vi "Read Multiple Sequence.vi"(6 "Segment number (0: All segment)":i16, 8 "error in (no error)":errorcluster, 9 "Timeout (10000 ms)":u32=10000, 10 "Channels":u16[](array[ring])=[0, 1] items=["Channel 1", "Channel 2", "Channel 3", "Channel 4", "Memory 1", "Memory 2", "Memory 3", "Memory 4", "Function 1", "Function 2", "Function 3", "Function 4", "Function 5", "Function 6", "Function 7", "Function 8"], 11 "VISA resource name":refnum<visa-resource-name>) -> (0 "error out":errorcluster, 2 "Waveform Data":waveform(dbl)[](graph), 3 "VISA resource name out":refnum<visa-resource-name>)   [LabVIEW 2013, in "LeCroy Wave Series.lvlib"]
doc: "Initiates an acquisition on all channels that you enabled with the <B>Configure Channel</B> VI. The VI waits for the acquisition to complete and returns the segments of waveform for the Source Channels you specified. If the oscilloscope did not complete the acquisition within the time period you specify with the Timeout parameter, the VI returns a time out error. A common cause for a timeout error is the acquisition was not triggered. For example, the trigger level is out of range of the waveform. \n\nNote: If your instrument does not support auto compensation for probe attenuation, you may need to adjust the scaling of the Waveform Data accordingly. This is handled automatically in the <B>Configure Channel</B> VI or can be done manually by multiplying the Waveform Data by the probe attenuation."
uses:
  LeCroy Wave Series.lvlib
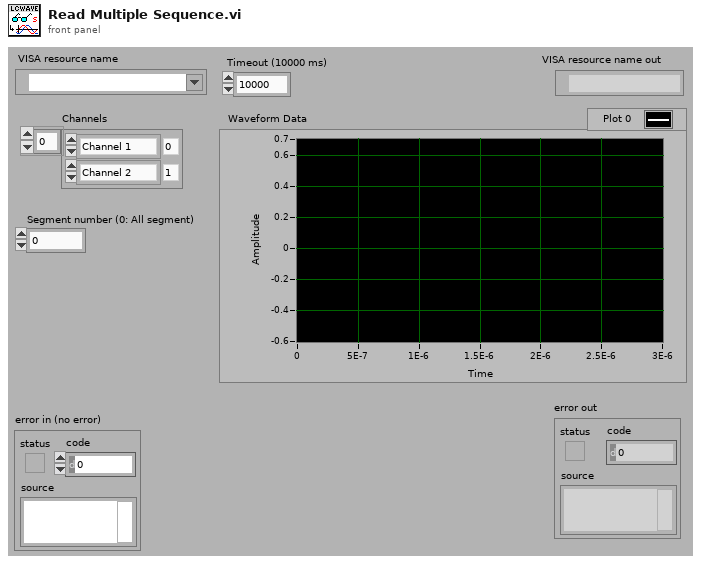
[diagram p1: front panel]
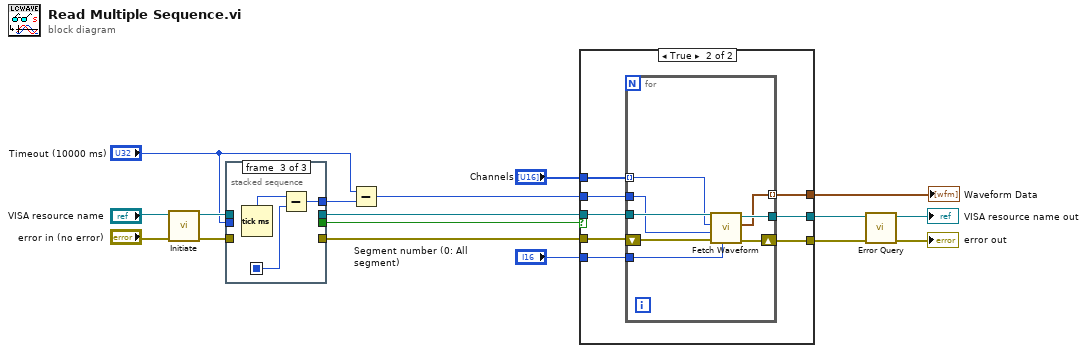
[diagram p0: block diagram]
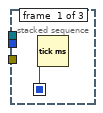
[diagram p2: hidden frame]
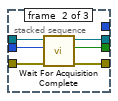
[diagram p3: hidden frame]
diagram:
  n1 = call "Initiate.vi"("error in (no error)"="error in (no error)", "VISA resource name"="VISA resource name") -> ("error out"=w12:errorcluster, "VISA resource name out"=w13:refnum<visa-resource-name>)  [unwired: 8 in]
  n2 = stacked-sequence {
    seq-local: [w18 _ _] -> [_ _ w26]
    tunnel: "Timeout (10000 ms)" -> [_ w24 _]
    tunnel: w13 -> [_ w22 _]
    tunnel: w12 -> [_ w20 _]
    tunnel: [_ w19 _] -> w11
    tunnel: [_ w21 _] -> w10
    tunnel: [_ _ w25] -> w14
    tunnel: [_ w23 _] -> w9
    frame #0 {
      n3 = Tick Count (ms)() -> (millisecond timer value=w18:u32)
    }
    frame #1 {
      n4 = call "Wait For Acquisition Complete.vi"("error in (no error)"=w20, "Timeout (10000 ms)"=w24, "VISA resource name"=w22) -> ("error out"=w19:errorcluster, "Complete"=w23:bool, "VISA resource name out"=w21:refnum<visa-resource-name>)  [unwired: 6 in]
    }
    frame #2 {
      n5 = Tick Count (ms)() -> (millisecond timer value=w27:u32)
      n6 = Subtract(x=w27, y=w26) -> (x-y=w25:u32)
    }
  }
  n7 = Subtract(x="Timeout (10000 ms)", y=w14) -> (x-y=w7:u32)
  n8 = case shown="True" w9 {
    tunnel: [_ w37] -> w15
    tunnel: [w29 w36] -> w6
    tunnel: [w28 w35] -> w4
    tunnel: w11 -> [w28 w34]
    tunnel: w10 -> [w29 w33]
    tunnel: w7 -> [_ w32]
    tunnel: "Channels" -> [_ w31]
    tunnel: "Segment number (0: All segment)" -> [_ w30]
    frame False {
    }
    frame True {
      n9 = for {
        tunnel: [w45] -> w36
        tunnel: w33 -> [w43]
        shift-right: [w44] -> w35
        shift-left: w34 -> [w42]
        tunnel: [w41] -> w37 mode=indexing
        tunnel: w32 -> [w38]
        tunnel: w31 -> [w40] mode=indexing
        tunnel: w30 -> [w39]
        n10 = call "Fetch Waveform.vi"("Segment number (0: All segment)"=w39, "error in (no error)"=w42, "Timeout (10000 ms)"=w38, "Source (0: Channel 1)"=w40, "VISA resource name"=w43) -> ("error out"=w44:errorcluster, "Waveform Graph"=w41:waveform(dbl), "VISA resource name out"=w45:refnum<visa-resource-name>)  [unwired: 4 in]
      }
    }
  }
  "Waveform Data" <- w15
  n11 = call "Error Query.vi"("error in (no error)"=w4, "VISA resource name"=w6) -> ("error out"=→"error out":errorcluster, "VISA resource name out"=→"VISA resource name out":refnum<visa-resource-name>)  [unwired: 6 in, 2 out]
